vi "SetAttribute.vi"(8 "error in (no error)":errorcluster, 10 "Set Attribute":T1, 11 "Data_General in":refnum<class "Data_FrameInfo.lvclass">) -> (0 "error out":errorcluster, 3 "Data_General out":refnum<class "Data_FrameInfo.lvclass">)   [LabVIEW 2020, in "Data_FrameInfo.lvclass"]
uses:
  Data_FrameInfo.lvclass
  Attribute.vi
  Data_FrameInfo.lvclass/Data_FrameInfo.ctl
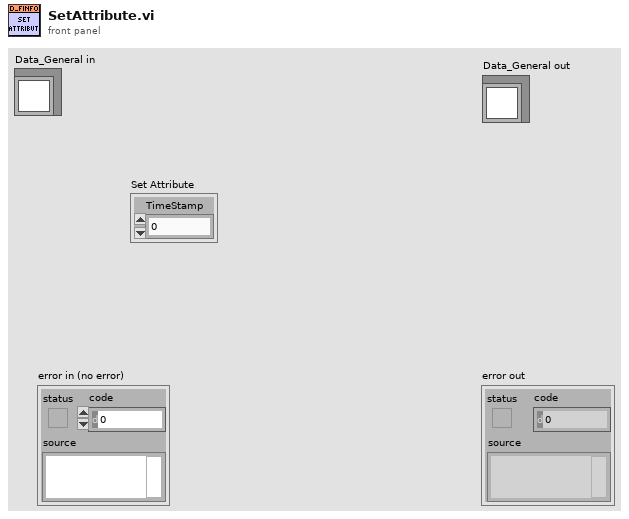
[diagram p1: front panel]
types:
  T1 = typedef "Data_FrameInfo.lvclass/Attribute.vi" = cluster{"TimeStamp":u64}
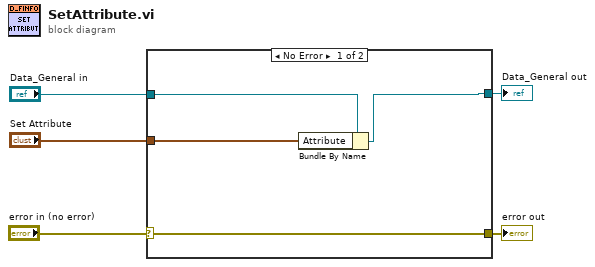
[diagram p0: block diagram]
diagram:
  n1 = case shown="No Error" "error in (no error)" {
    selector: "error in (no error)" -> [w9 w11]
    tunnel: [w9 w11] -> w4
    tunnel: [w7 w10] -> w3
    tunnel: "Data_General in" -> [w8 w10]
    tunnel: "Set Attribute" -> [w6 _]
    frame No Error {
      n2 = Bundle By Name(cluster=w8, "Attribute"=w6) -> (w7:refnum<class "Data_FrameInfo.lvclass">)
    }
    frame Error {
    }
  }
  "error out" <- w4
  "Data_General out" <- w3
